vi "Cam prepare buffer.vi"(8 "error in (no error)":errorcluster, 11 "Camera in":refnum<class "Camera.lvclass">) -> (0 "error out":errorcluster, 3 "Camera out":refnum<class "Camera.lvclass">)   [LabVIEW 2021, in "Camera.lvlib" / "Camera.lvclass"]
uses:
  Camera.lvclass
  Camera.lvclass/Camera.ctl
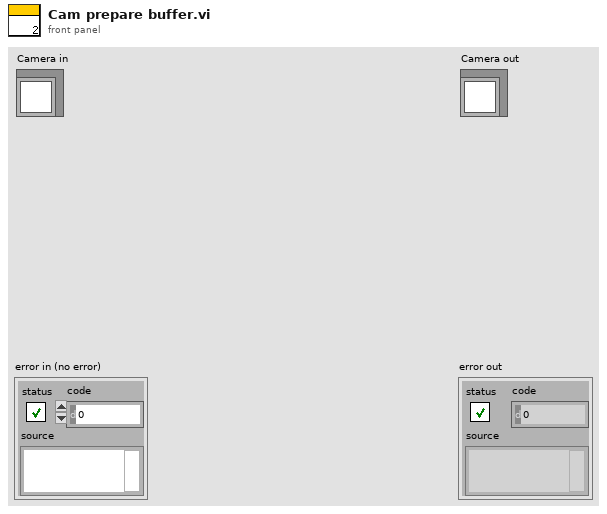
[diagram p1: front panel]
types:
  T1 = typedef "IMAQ Image.ctl" = refnum<image>
  T2 = typedef "Camera.lvlib/Camera.lvclass/Cam task parameters.ctl" = cluster{"exposure time":dbl, "camera W":dbl, "camera H":dbl, "y line #":dbl, "flyback line #":dbl, "buffer page#":dbl, "frame#":dbl}
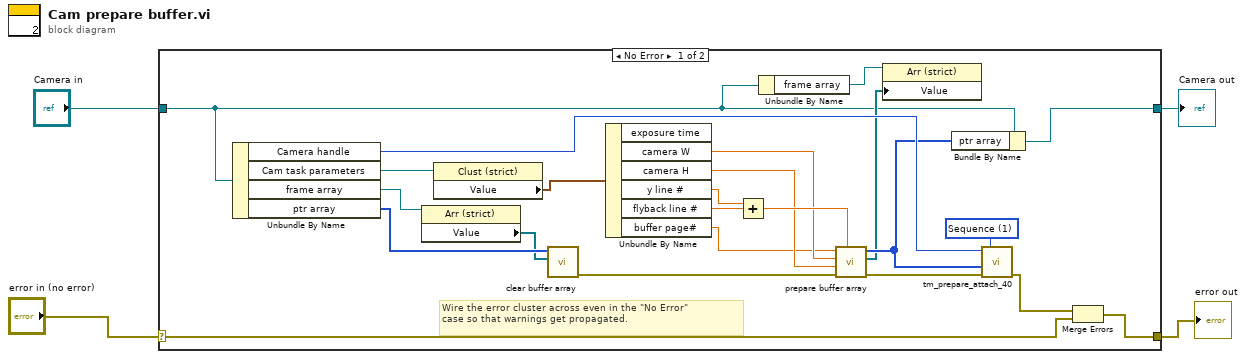
[diagram p0: block diagram]
diagram:
  n1 = case shown="No Error" "error in (no error)" {
    selector: "error in (no error)" -> [w6 w29]
    tunnel: [w5 w29] -> w3
    tunnel: [w19 w28] -> w1
    tunnel: "Camera in" -> [w9 w28]
    frame No Error {
      w16 = 1 items=["Snap", "Sequence"] ("Capture mode")
      # "Wire the error cluster across even in the \"No Error\"\ncase so that warnings get propagated."
      n2 = Unbundle By Name(w9) -> ("Camera handle"=w17:u32, "Cam task parameters"=w14:refnum<vi>, "frame array"=w12:refnum<vi>, "ptr array"=w27:u64[])
      n3 = property class="Arr (strict)"(reference=w12) -> ("Value"=w11:T1[])  [unwired: 1 in, 2 out]
      n4 = property class="Clust (strict)"(reference=w14) -> ("Value"=w13:T2)  [unwired: 1 in, 2 out]
      n5 = call "clear buffer array.vi"("Image array"=w11, "ptr array"=w27) -> ("error out"=w26:errorcluster)  [unwired: 9 in]
      n6 = Unbundle By Name(w13) -> ("camera W"=w22:dbl, "camera H"=w21:dbl, "y line #"=w24:dbl, "flyback line #"=w25:dbl, "buffer page#"=w20:dbl)  [unwired: 1 out]
      n7 = Add(x=w24, y=w25) -> (x+y=w23:dbl)
      n8 = Unbundle By Name(w9) -> ("frame array"=w8:refnum<vi>)
      n9 = call "prepare buffer array.vi"("shots# per page"=w23, "error in (no error)"=w26, "shot H"=w21, "page W"=w22, "buffer page #"=w20) -> ("error out"=w18:errorcluster, "Image array"=w10:T1[], "ptr array"=w15:u64[])  [unwired: 4 in]
      n10 = property class="Arr (strict)"(reference=w8, "Value"=w10) -> ()  [unwired: 1 in, 2 out]
      n11 = Bundle By Name(cluster=w9, "ptr array"=w15) -> (w19:refnum<class "Camera.lvclass">)
      n12 = call <userlib>:"tm_prepare_attach_40.vi"("error in (no error)"=w18, "buffers"=w15, "Capture mode"=w16, "Handle in"=w17) -> ("error out"=w7:errorcluster)  [unwired: 6 in, 1 out]
      n13 = Merge Errors(w7, w6) -> (w5:errorcluster)
    }
    frame Error {
    }
  }
  "error out" <- w3
  "Camera out" <- w1
